vi "testDriver.vi"() -> ()   [LabVIEW 2012]
uses:
  <vilib>/DAQmx/configure/timing.llb/DAQmx Timing (Implicit).vi
  <resource>/objmgr/daqmx.rc
panel:
  out "Boolean":bool
  in  "stop":bool
  out "pulse 1/2 len (ms)":dbl
  in  "Meter":dbl(knob) scale=0.0..49.0
  out "mm/s (timed)":dbl
  in  "Run":bool
  in  "travel dist(mm)":i32=100
  in  "Direction":bool
  # "=17400 to go across"
  # "0.0001"
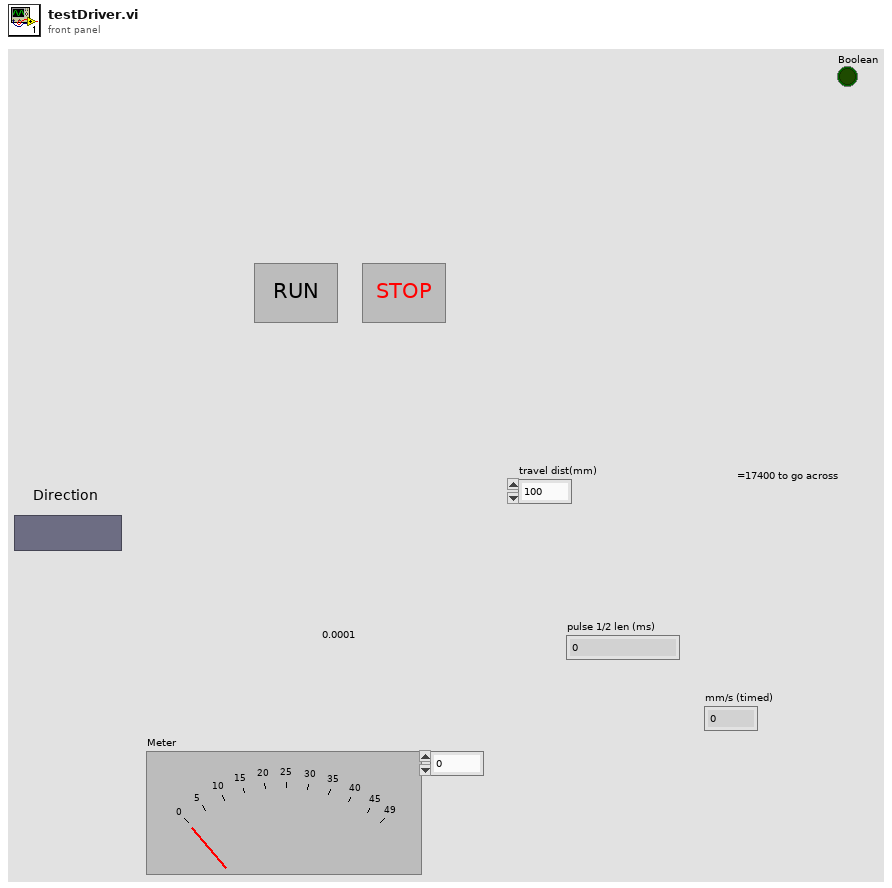
[diagram p1: front panel]
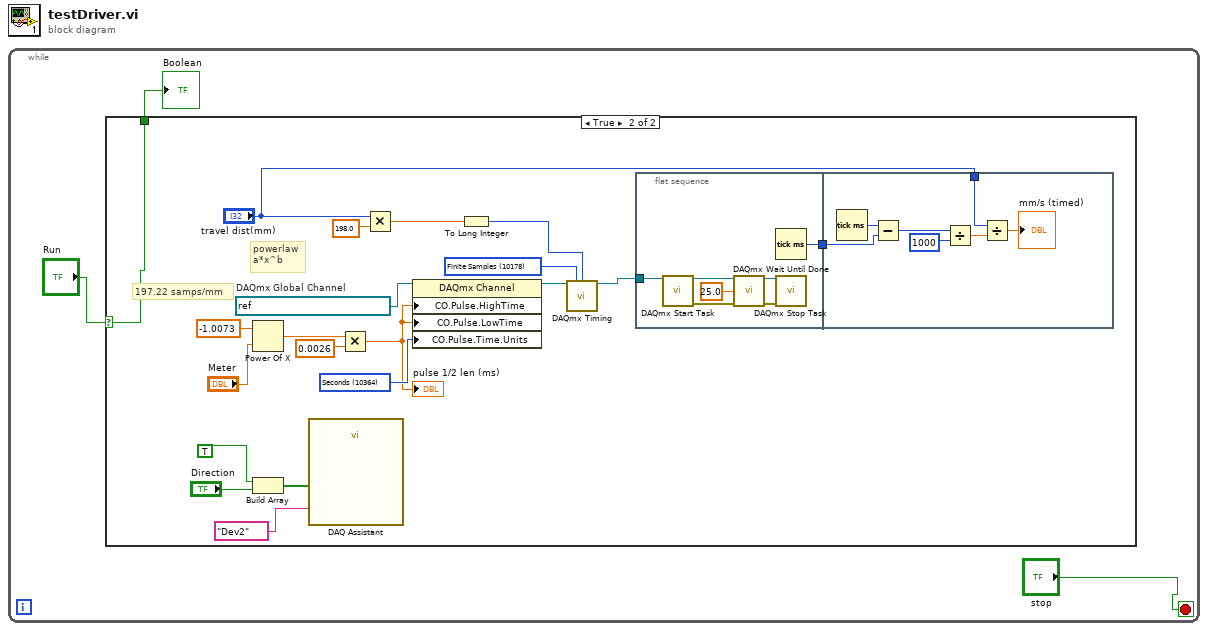
[diagram p0: block diagram]
diagram:
  n1 = while {
    stop <- "stop" stop-if-true
    n2 = case shown="True" "Run" {
      selector: "Run" -> [w4 w5]
      tunnel: [w4 w5] -> w1
      frame False {
      }
      frame True {
        w22 = 10364 items=["Seconds"=10364] ("CO.Pulse.Time.Units")
        w19 = 10178 items=["Finite Samples"=10178, "Continuous Samples"=10123, "Hardware Timed Single Point"=12522] ("sample mode")
        w18 = refnum<k21> "MyPulseOutputChannel"  # DAQmx Global Channel
        # "powerlaw\na*x^b"
        # "197.22 samps/mm"
        n3 = Power Of X(1:"Meter", 2:-1.0073) -> (0:w9:dbl)
        n4 = Build Array(TRUE ("element"), "Direction") -> (w16:bool[])
        n5 = call "DAQ Assistant"("data"=w16, "device name"=tag "Dev2") -> ()  [unwired: 16 in, 2 out]
        n6 = Multiply(x=w9, y=0.0026) -> (x*y=w7:dbl)
        "pulse 1/2 len (ms)" <- w7
        n7 = Multiply(x="travel dist(mm)", y=198.0) -> (x*y=w14:dbl)
        n8 = property class="DAQmx Channel"(reference=w18, "CO.Pulse.HighTime"=w7, "CO.Pulse.LowTime"=w7, "CO.Pulse.Time.Units"=w22) -> (reference out=w21:refnum<k21>)  [unwired: 1 in, 1 out]
        n9 = To Long Integer(number=w14) -> (32bit integer=w13:i32)
        n10 = call-poly <vilib>:"DAQmx Timing.vi"("task/channels in"=w21, "sample mode"=w19, "samples per channel"=w13) -> ("task out"=w20:refnum<k21>)  [unwired: 11 in, 1 out]
        n11 = flat-sequence {
          tunnel: w20 -> [w29]
          tunnel: [w25] -> w24
          tunnel: w24 -> [w38]
          tunnel: "travel dist(mm)" -> [w34]
          frame #0 {
            n12 = call <vilib>:"DAQmx Start Task.vi"("task/channels in"=w29) -> ("task out"=w30:refnum<k21>, "error out"=w27:errorcluster)  [unwired: 13 in]
            n13 = call <vilib>:"DAQmx Wait Until Done.vi"("task/channels in"=w30, "timeout (sec)"=25.0, "error in"=w27) -> ("task out"=w28:refnum<k21>, "error out"=w26:errorcluster)  [unwired: 11 in]
            n14 = Tick Count (ms)() -> (millisecond timer value=w25:u32)
            n15 = call <vilib>:"DAQmx Stop Task.vi"("task/channels in"=w28, "error in"=w26) -> ()  [unwired: 12 in, 2 out]
          }
          frame #1 {
            n16 = Tick Count (ms)() -> (millisecond timer value=w37:u32)
            n17 = Subtract(x=w37, y=w38) -> (x-y=w36:u32)
            n18 = Divide(x=w36, y=u32 1000) -> (x/y=w33:dbl)
            n19 = Divide(x=w34, y=w33) -> (x/y=→"mm/s (timed)":dbl)
          }
        }
      }
    }
    "Boolean" <- w1
  }
